vi "top level vi.vi"() -> ()   [LabVIEW 2014]
panel:
  out "last 5 temp":dbl(graph)
  out "current Temp":dbl(graph)
  in  "y":dbl
  in  "x":dbl
  in  "stop":bool
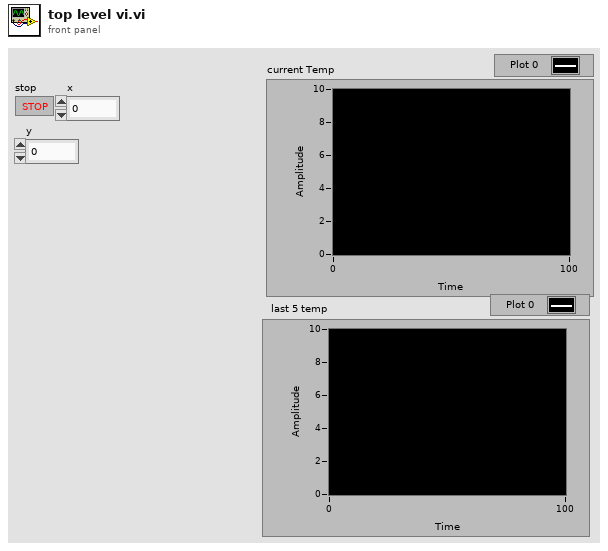
[diagram p1: front panel]
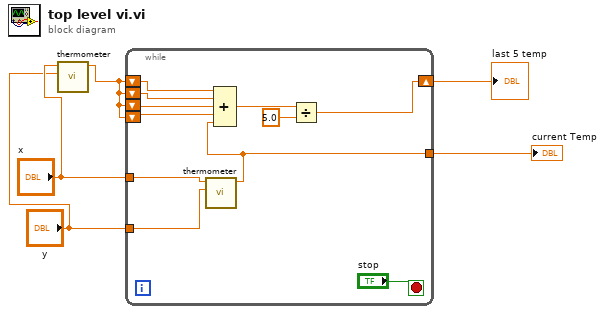
[diagram p0: block diagram]
diagram:
  n1 = call "thermometer.vi"("y"="y", "x"="x") -> ("Numeric"=w2:dbl)  [unwired: 9 in]
  n2 = while {
    tunnel: [w9] -> w5
    tunnel: "x" -> [w15]
    tunnel: "y" -> [w14]
    shift-right: [w6] -> w1
    shift-left: w2 -> [w13]
    shift-left: w2 -> [w12]
    shift-left: w2 -> [w11]
    shift-left: w2 -> [w10]
    stop <- "stop" stop-if-true
    n3 = call "thermometer.vi"("y"=w14, "x"=w15) -> ("Numeric"=w9:dbl)  [unwired: 9 in]
    n4 = Compound Arithmetic op=ADD(w13, w12, w11, w10, w9) -> (w8:dbl)
    n5 = Divide(x=w8, y=5.0) -> (x/y=w6:dbl)
  }
  "current Temp" <- w5
  "last 5 temp" <- w1
